vi "MRC Console Write Program Crash.vi"(8 "error in (no error)":errorcluster, 9 "stackTrace":T1, 10 "location":T1, 11 "message":T1) -> (0 "error out":errorcluster)   [LabVIEW 2026, in "MrcLib.lvlib"]
doc: "MRC_Status MRC_CALLCONV MRC_Console_WriteProgramCrash(\n const struct MRC_String* message, const struct MRC_String* location,\n const struct MRC_String* stackTrace);"
uses:
  MrcLib.lvlib
  <vilib>/MRC/Types/MRC String.ctl
  MrcLib.dll
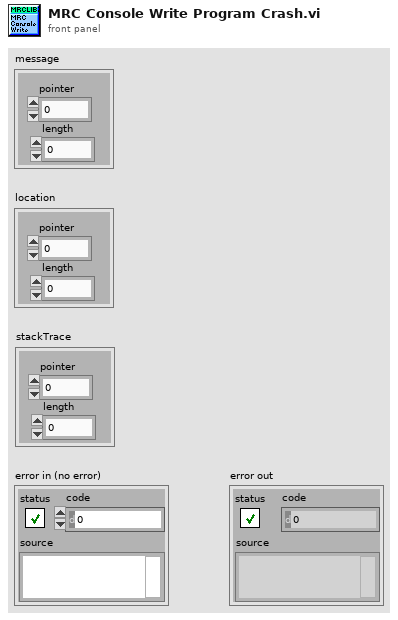
[diagram p1: front panel]
types:
  T1 = typedef "MRC String.ctl" = cluster{"pointer":u64, "length":u64}
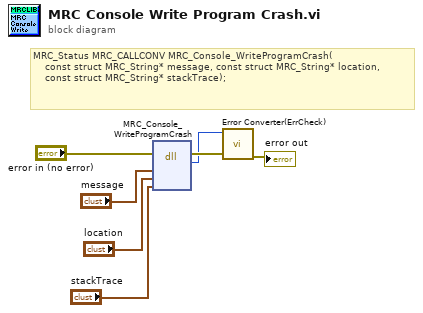
[diagram p0: block diagram]
diagram:
  # "MRC_Status MRC_CALLCONV MRC_Console_WriteProgramCrash(\n    const struct MRC_String* message, const struct MRC_String* location,\n    const struct MRC_String* stackTrace);"
  n1 = dll-call lib="MrcLib.*" fn="MRC_Console_WriteProgramCrash"(error in="error in (no error)", "message"="message", "location"="location", "stackTrace"="stackTrace") -> (error out=w3:errorcluster, "return type"=w1:i32)  [unwired: 5 in, 1 out]
  n2 = call <vilib>:"Error Converter(ErrCheck).vi"("error in (no error)"=w3, "status"=w1) -> ("error out"=→"error out":errorcluster)  [unwired: 9 in]
